vi "5302GPIBComm.vi"(8 "error in (no error)":errorcluster, 9 "data string in":string, 10 "address":i16) -> (0 "error out":errorcluster, 1 "data string out":string)   [LabVIEW 2015]
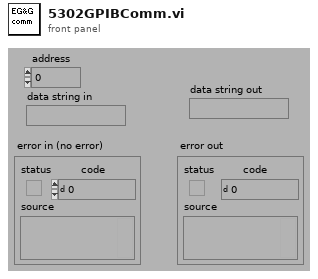
[diagram p1: front panel]
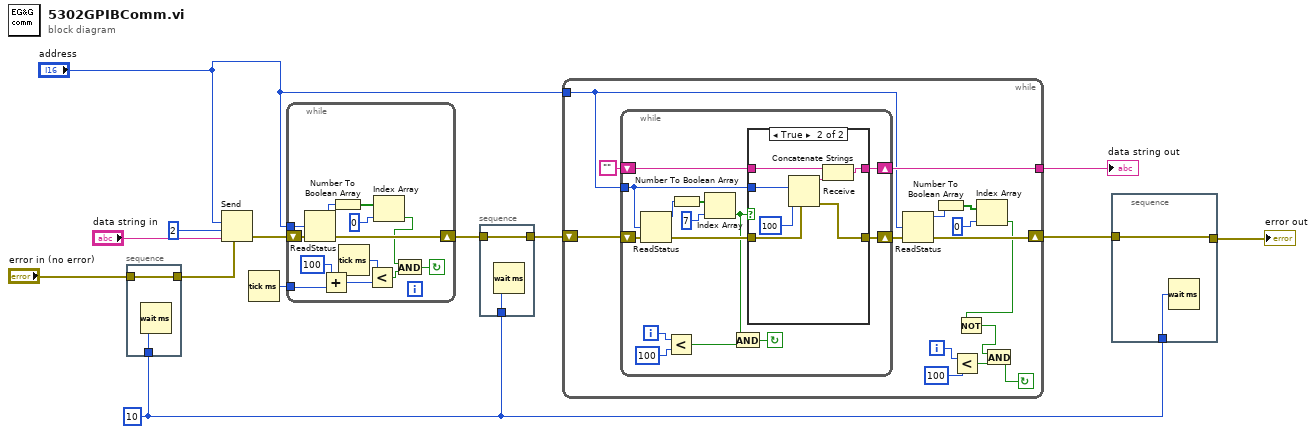
[diagram p0: block diagram]
diagram:
  w1 = 10
  n1 = stacked-sequence {
    tunnel: "error in (no error)" -> [w15]
    tunnel: [w15] -> w4
    tunnel: w1 -> [w14]
    frame #0 {
      n2 = Wait (ms)(milliseconds to wait=w14) -> ()  [unwired: 1 out]
    }
  }
  n3 = Send(2:"address", 3:i16 2 ("mode"), 4:w4, 5:"data string in") -> (8:w11:errorcluster)  [unwired: 1 in, 2 out]
  n4 = Tick Count (ms)() -> (millisecond timer value=w9:u32)
  n5 = while {
    tunnel: "address" -> [w27]
    shift-right: [w26] -> w3
    shift-left: w11 -> [w28]
    tunnel: w9 -> [w18]
    stop <- w25 continue-if-true
    n6 = ReadStatus(3:w28, 4:w27) -> (0:w26:errorcluster, 2:w21:i16)  [unwired: 1 in, 1 out]
    n7 = Add(x=u32 100, y=w18) -> (x+y=w19:u32)
    n8 = Number To Boolean Array(number=w21) -> (Boolean array=w22:bool[])
    n9 = Tick Count (ms)() -> (millisecond timer value=w16:u32)
    n10 = Less?(x=w16, y=w19) -> (x < y?=w24:bool)
    n11 = Index Array(array=w22, index=0) -> (element=w20:bool)
    n12 = And(x=w20, y=w24) -> (x .and. y?=w25:bool)
  }
  n13 = stacked-sequence {
    tunnel: w3 -> [w30]
    tunnel: [w30] -> w2
    tunnel: w1 -> [w29]
    frame #0 {
      n14 = Wait (ms)(milliseconds to wait=w29) -> ()  [unwired: 1 out]
    }
  }
  n15 = while {
    tunnel: "address" -> [w40]
    tunnel: [w42] -> w10
    shift-right: [w41] -> w7
    shift-left: w2 -> [w45]
    i -> [w35]
    stop <- w33 continue-if-true
    n16 = while {
      tunnel: w40 -> [w55]
      shift-right: [w54] -> w43
      shift-left: w45 -> [w59]
      shift-right: [w53] -> w42
      shift-left: "" -> [w52]
      i -> [w51]
      stop <- w58 continue-if-true
      n17 = ReadStatus(3:w59, 4:w55) -> (0:w56:errorcluster, 2:w47:i16)  [unwired: 1 in, 1 out]
      n18 = Less?(x=w51, y=100 ("x")) -> (x < y?=w57:bool)
      n19 = Number To Boolean Array(number=w47) -> (Boolean array=w49:bool[])
      n20 = Index Array(array=w49, index=7) -> (element=w46:bool)
      n21 = And(x=w46, y=w57) -> (x .and. y?=w58:bool)
      n22 = case shown="True" w46 {
        tunnel: w56 -> [w61 w67]
        tunnel: w55 -> [_ w65]
        tunnel: [w61 w66] -> w54
        tunnel: [w60 w63] -> w53
        tunnel: w52 -> [w60 w62]
        frame False {
        }
        frame True {
          n23 = Receive(4:w67, 6:100 ("count"), 8:w65) -> (0:w66:errorcluster, 3:w64:string)  [unwired: 2 in, 2 out]
          n24 = Concatenate Strings(w62, w64) -> (w63:string)
        }
      }
    }
    n25 = ReadStatus(3:w43, 4:w40) -> (0:w41:errorcluster, 2:w37:i16)  [unwired: 1 in, 1 out]
    n26 = Number To Boolean Array(number=w37) -> (Boolean array=w38:bool[])
    n27 = Less?(x=w35, y=100 ("x")) -> (x < y?=w34:bool)
    n28 = Index Array(array=w38, index=0) -> (element=w31:bool)
    n29 = Not(x=w31) -> (.not. x?=w32:bool)
    n30 = And(x=w32, y=w34) -> (x .and. y?=w33:bool)
  }
  "data string out" <- w10
  n31 = stacked-sequence {
    tunnel: [w70] -> w8
    tunnel: w7 -> [w70]
    tunnel: w1 -> [w69]
    frame #0 {
      n32 = Wait (ms)(milliseconds to wait=w69) -> ()  [unwired: 1 out]
    }
  }
  "error out" <- w8
